vi "HandleClapper.vi"(7 "InitState":T1=enum."Middle", 8 "error in (no error)":errorcluster, 11 "Toggle?":bool) -> (0 "error out":errorcluster, 3 "State":T1)   [LabVIEW 2013]
uses:
  DoubleSolenoidAction.ctl
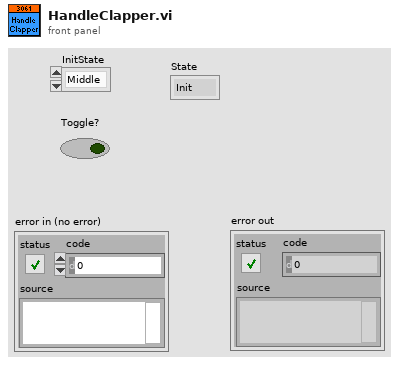
[diagram p1: front panel]
types:
  T1 = typedef "DoubleSolenoidAction.ctl" = enum16{"Init", "Middle", "In", "Out"}
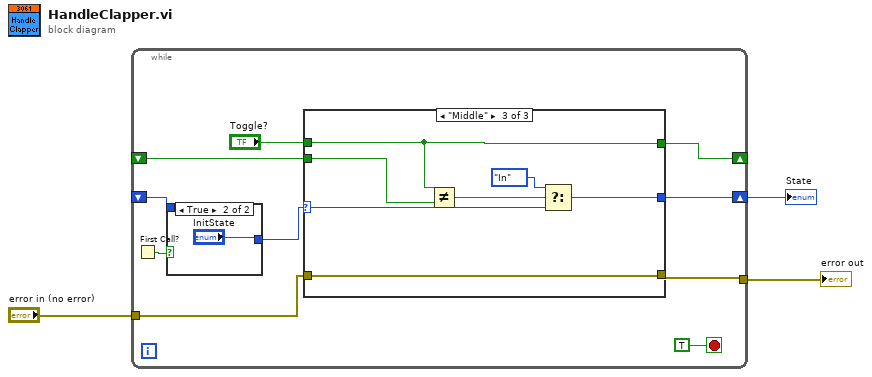
[diagram p0: block diagram]
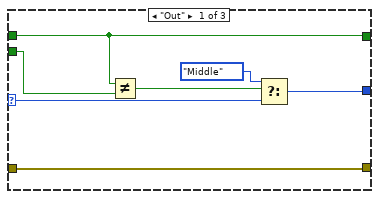
[diagram p3: hidden frame]
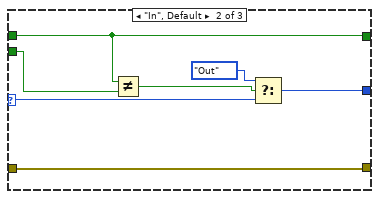
[diagram p4: hidden frame]
diagram:
  n1 = while {
    shift-right: [w12] -> w3
    shift-left: _ -> [w9]
    shift-right: [w7] -> _
    shift-left: _ -> [w6]
    tunnel: "error in (no error)" -> [w5]
    tunnel: [w4] -> w1
    stop <- TRUE stop-if-true
    n2 = First Call?() -> (First Call?: T/F=w11:bool)
    n3 = case shown="True" w11 {
      tunnel: [w14 "InitState"] -> w10
      tunnel: w9 -> [w14 _]
      frame False {
      }
      frame True {
      }
    }
    n4 = case shown="\"Middle\"" w10 {
      selector: w10 -> [w20 w27 w36]
      tunnel: [w21 w28 w35] -> w12
      tunnel: [w17 w25 w33] -> w7
      tunnel: "Toggle?" -> [w17 w25 w33]
      tunnel: w6 -> [w18 w24 w32]
      tunnel: w5 -> [w16 w23 w30]
      tunnel: [w16 w23 w30] -> w4
      frame "Out" {
        n5 = Not Equal?(x=w17, y=w18) -> (x != y?=w19:bool)
        n6 = Select(t=DoubleSolenoidAction."Middle", s=w19, f=w20) -> (s? t:f=w21:T1)
      }
      frame "In", Default {
        n7 = Not Equal?(x=w25, y=w24) -> (x != y?=w26:bool)
        n8 = Select(t=DoubleSolenoidAction."Out", s=w26, f=w27) -> (s? t:f=w28:T1)
      }
      frame "Middle" {
        n9 = Not Equal?(x=w33, y=w32) -> (x != y?=w31:bool)
        n10 = Select(t=DoubleSolenoidAction."In", s=w31, f=w36) -> (s? t:f=w35:T1)
      }
    }
  }
  "State" <- w3
  "error out" <- w1
